vi "Write_Digitals.vi"(0 "digitals to write":u64) -> (1 "Aborted":bool, 2 "Error Out":u8)   [LabVIEW 2017]
uses:
  <vilib>/rvi/eio/common/nirviEmuTemplateMethod_errors.vi
  <vilib>/rvi/Emulation/niFpgaEmulationIsFPGAContextNoSignature.vi
  <vilib>/rvi/DataTransferAndStorage/Container/Common/niFpgaContainerGetUniqueNameForEmu.vi
  <vilib>/rvi/Memory/Memory_Emulation/niFpgaMemoryEmulationCacheClearOnFirstRun.vi
  <vilib>/rvi/Memory/Memory_Emulation/nirvimemoryEmulationManagerCache_MakeExclusive.vi
  <vilib>/rvi/Memory/Memory_Emulation/niFpgaMemoryEmulationValidateCache.vi
  <vilib>/rvi/Memory/Memory_Emulation/nirvimemoryEmulationManagerCache_InsertValue.vi
  <vilib>/Utility/error.llb/Clear Errors.vi
  <vilib>/rvi/Memory/Memory_Emulation/nirvimemoryEmulationManagerCache_ReleaseExclusive.vi
  <vilib>/rvi/Memory/Memory_Emulation/nirvimemoryEmulationManagerCache_GetValue.vi
  <vilib>/rvi/Memory/Memory_Emulation/nirvimemoryEmulationManagerCache_SetValue.vi
  <vilib>/rvi/Emulation/niFpgaProcessEmulError.vi
  <vilib>/rvi/Emulation/niFpgaSctlEmulationGetInTimedLoop.vi
  <vilib>/eio/EIONode/EIONode.xnode
  <vilib>/rvi/DataTransferAndStorage/Container/XNode/niFpgaContainer.xnode
  <vilib>/rvi/DataTransferAndStorage/Register/Emulation/niFpgaRegisterEmulation.vi
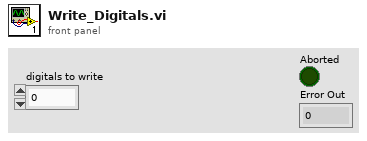
[diagram p1: front panel]
types:
  T1 = cluster{"Boolean array[0]":bool, "Boolean array[1]":bool, "Boolean array[2]":bool, "Boolean array[3]":bool, "Boolean array[4]":bool, "Boolean array[5]":bool, "Boolean array[6]":bool, "Boolean array[7]":bool, "Boolean array[8]":bool, "Boolean array[9]":bool, "Boolean array[10]":bool, "Boolean array[11]":bool, "Boolean array[12]":bool, "Boolean array[13]":bool, "Boolean array[14]":bool, "Boolean array[15]":bool}
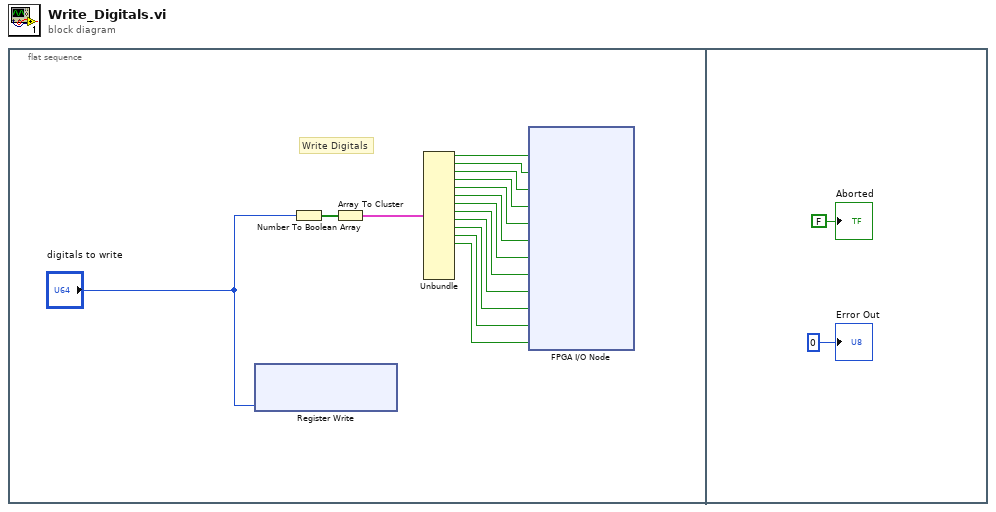
[diagram p0: block diagram]
diagram:
  n1 = flat-sequence {
    frame #0 {
      # "Write Digitals"
      n2 = xnode ("Register Write")("Data"="digitals to write") -> ()  [unwired: 1 in, 1 out]
      n3 = Number To Boolean Array(number="digitals to write") -> (Boolean array=w3:bool[])
      n4 = Array To Cluster(array=w3) -> (cluster=w2:T1)
      n5 = Unbundle(w2) -> ("Boolean array[0]"=w4:bool, "Boolean array[1]"=w5:bool, "Boolean array[2]"=w15:bool, "Boolean array[3]"=w14:bool, "Boolean array[4]"=w13:bool, "Boolean array[5]"=w12:bool, "Boolean array[6]"=w11:bool, "Boolean array[7]"=w10:bool, "Boolean array[8]"=w9:bool, "Boolean array[9]"=w8:bool, "Boolean array[10]"=w7:bool, "Boolean array[11]"=w6:bool)  [unwired: 4 out]
      n6 = xnode "FPGA I/O Node"("Mod2/DIO0"=w4, "Mod2/DIO1"=w5, "Mod2/DIO2"=w15, "Mod2/DIO3"=w14, "Mod3/DIO0"=w13, "Mod3/DIO1"=w12, "Mod3/DIO2"=w11, "Mod3/DIO3"=w10, "Mod4/DIO0"=w9, "Mod4/DIO1"=w8, "Mod4/DIO2"=w7, "Mod4/DIO3"=w6) -> ()  [unwired: 12 in, 12 out]
    }
    frame #1 {
      "Aborted" <- FALSE
      "Error Out" <- u8 0
    }
  }
